vi "testRPM3.vi"() -> ()   [LabVIEW 2014]
uses:
  <vilib>/measure/NI_MAPro.lvlib
  <vilib>/measure/mamon.llb/Trigger Detection for 1 Channel.vi
panel:
  out "Boolean":bool
  in  "Histerese":dbl
  in  "Level":dbl
  in  "Fator":dbl
  out "Velocidade(km_h)":u8
  out "RPM":dbl
  out "Frequency (RPM)":dbl
  out "Filtered Signal 2":dynamicdata(graph) caption="Filtered Signal"
  out "error out":errorcluster
  in  "stop":bool
  out "Frequency":dbl
  out "Raw Signal":dynamicdata(graph) caption="Filtered Signal"
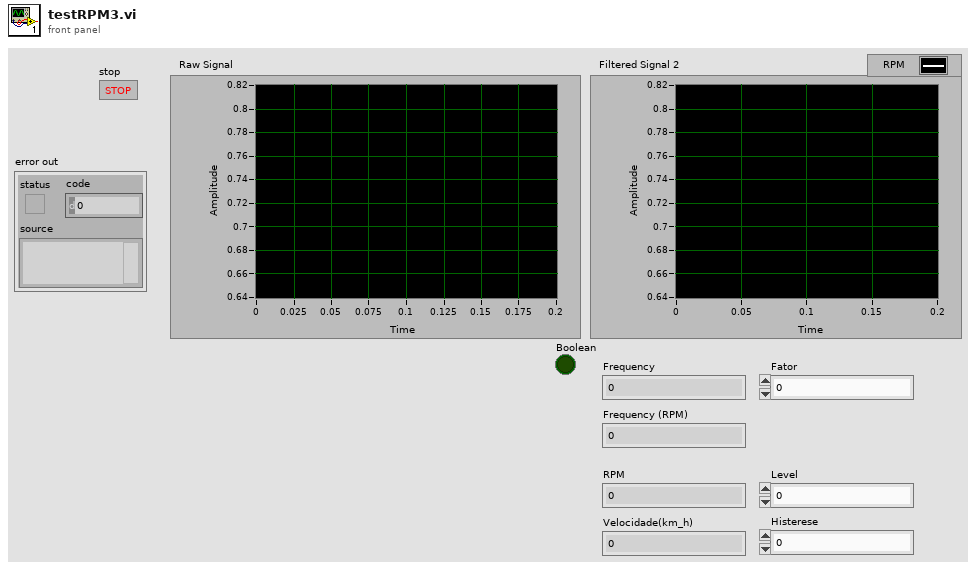
[diagram p1: front panel]
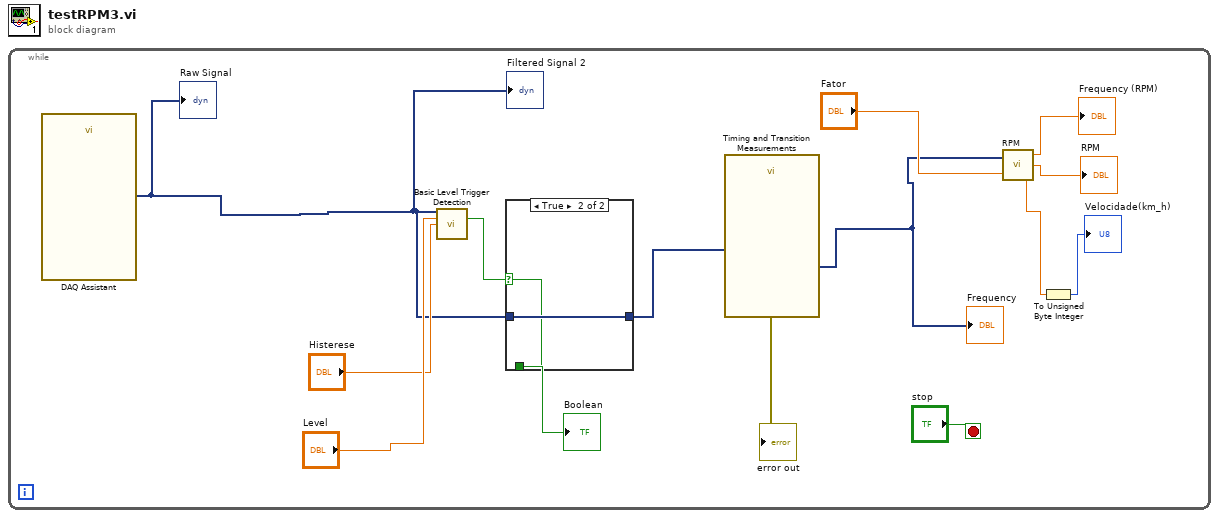
[diagram p0: block diagram]
diagram:
  n1 = while {
    stop <- "stop" stop-if-true
    n2 = call "DAQ Assistant"() -> ("data"=w3:dynamicdata)  [unwired: 16 in, 3 out]
    "Raw Signal" <- w3
    "Filtered Signal 2" <- w3
    n3 = call-poly <vilib>:"Basic Level Trigger Detection.vi"("signal in"=w3, "level"="Level", "hysteresis"="Histerese") -> ("trigger detected?"=w9:bool)  [unwired: 10 in, 2 out]
    n4 = case shown="True" w9 {
      selector: w9 -> [w15 w16]
      tunnel: w3 -> [_ w17]
      tunnel: [_ w17] -> w8
      tunnel: [w15 w16] -> w6
      frame False {
      }
      frame True {
      }
    }
    "Boolean" <- w6
    n5 = call "Timing and Transition Measurements"("Signals"=w8) -> ("error out"=→"error out":errorcluster, "Frequency"=w7:dynamicdata)  [unwired: 9 in]
    "Frequency" <- w7
    n6 = call "RPM.vi"("data"=w7, "factor"="Fator") -> ("Frequency"=→"Frequency (RPM)":dbl, "RPM"=→"RPM":dbl, "km/h"=w2:dbl)
    n7 = To Unsigned Byte Integer(number=w2) -> (unsigned 8bit integer=→"Velocidade(km_h)":u8)
  }
